vi "Copy .LLB to NI VeriStand dir.vi"(5 "Files Generated by Build":path[](array[path]), 6 "Top Level/Always Included VIs":path[](array[path]), 7 "Destination Path":path, 8 "error in (no error)":errorcluster, 9 "Target Name":string, 10 "Build Specification Name":string, 11 "Project Path":path) -> (0 "error out":errorcluster)   [LabVIEW 2015]
doc: "This VI is called after each run of a build specification. The VI will copy the generated LLB (Engine or System Explorer) into the VeriStand Custom Device folder (...\\Documents\\National Instruments\\NI VeriStand 2013...)."
uses:
  <vilib>/Utility/sysdir.llb/System Directory Type.ctl
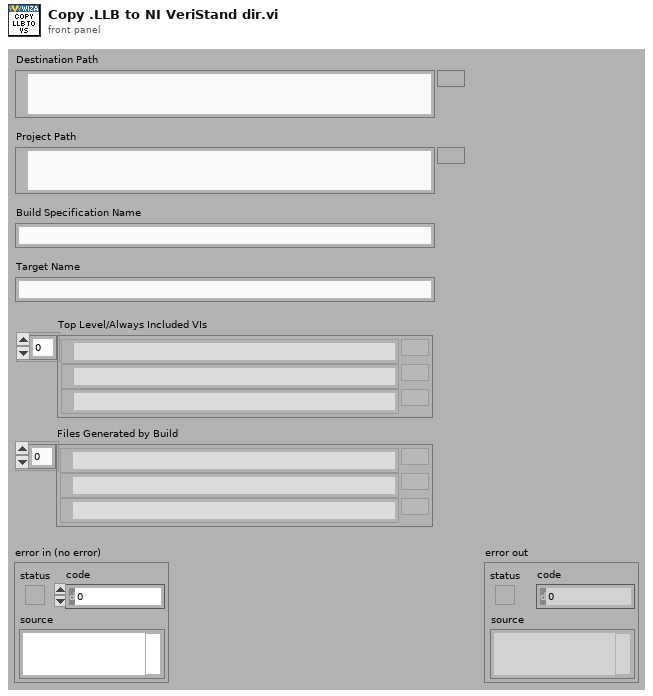
[diagram p1: front panel]
types:
  T1 = typedef "System Directory Type.ctl" = i32
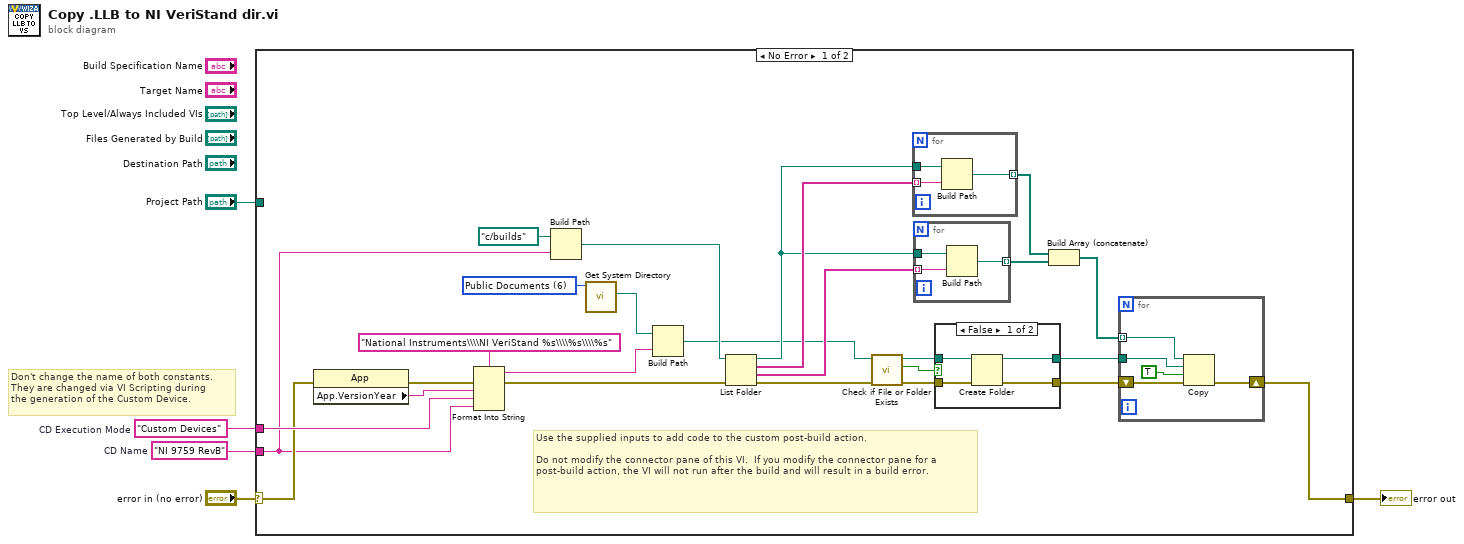
[diagram p0: block diagram]
diagram:
  w2 = "NI 9759 RevB"  # CD Name
  w3 = "Custom Devices"  # CD Execution Mode
  # "Don't change the name of both constants.\nThey are changed via VI Scripting during\nthe generation of the Custom Device."
  n1 = case shown="No Error" "error in (no error)" {
    selector: "error in (no error)" -> [w11 w49]
    tunnel: [w14 w49] -> w1
    tunnel: "Project Path" -> [_ _]
    tunnel: w3 -> [w12 _]
    tunnel: w2 -> [w9 _]
    frame No Error {
      w18 = T1 6 items=["User Home"=0, "User Desktop"=1, "User Documents"=2, "User Application Data"=3, "User Preferences"=4, "User Temporary"=5, "Public Documents"=6, "Public Application Data"=7, "Public Preferences"=8, "Public Cache"=13, "System Core Libraries"=9, "System Installed Libraries"=10, "Application Files"=11, "Boot Volume Root"=12] ("system directory type")
      # "Use the supplied inputs to add code to the custom post-build action.\n\nDo not modify the connector pane of this VI.  If you modify the connector pane for a post-build action, the VI will not run after the build and will result in a build error."
      n2 = property class="App"(error in=w11) -> (error out=w17:errorcluster, "App.VersionYear"=w16:string)  [unwired: 1 in, 1 out]
      n3 = Format Into String(format string="National Instruments\\\\NI VeriStand %s\\\\%s\\\\%s" ("name or relative path"), error in=w17, w16, w12, w9) -> (resulting string=w20:string, error out=w10:errorcluster)  [unwired: 1 in]
      n4 = Build Path(base path=path "c:/builds" ("name or relative path"), name or relative path=w9) -> (appended path=w22:path)
      n5 = call <vilib>:"Get System Directory.vi"("system directory type"=w18) -> ("system directory"=w19:path)  [unwired: 10 in]
      n6 = Build Path(base path=w19, name or relative path=w20) -> (appended path=w13:path)
      n7 = List Folder(path=w22, error in=w10) -> (path out=w24:path, filenames=w31:string[], folder names=w25:string[], error out=w21:errorcluster)  [unwired: 2 in]
      n8 = call <vilib>:"Check if File or Folder Exists.vi"("error in (no error)"=w21, "path"=w13) -> ("error out"=w26:errorcluster, "file or folder exists?"=w28:bool, "dup path"=w27:path)  [unwired: 7 in]
      n9 = for {
        tunnel: w31 -> [w47] mode=indexing
        tunnel: w24 -> [w48]
        tunnel: [w46] -> w30 mode=indexing
        n10 = Build Path(base path=w48, name or relative path=w47) -> (appended path=w46:path)
      }
      n11 = for {
        tunnel: w25 -> [w44] mode=indexing
        tunnel: w24 -> [w45]
        tunnel: [w43] -> w23 mode=indexing
        n12 = Build Path(base path=w45, name or relative path=w44) -> (appended path=w43:path)
      }
      n13 = case shown="False" w28 {
        tunnel: w27 -> [w35 w37]
        tunnel: w26 -> [w34 w36]
        tunnel: [w33 w37] -> w8
        tunnel: [w32 w36] -> w7
        frame False {
          n14 = Create Folder(path (use dialog)=w35, error in=w34) -> (created path=w33:path, error out=w32:errorcluster)  [unwired: 1 in, 1 out]
        }
        frame True {
        }
      }
      n15 = Build Array (concatenate)(w30, w23) -> (w29:path[])
      n16 = for {
        tunnel: w29 -> [w39] mode=indexing
        shift-right: [w40] -> w14
        shift-left: w7 -> [w41]
        tunnel: w8 -> [w38]
        n17 = Copy(8:w41, 9:TRUE ("overwrite (F)"), 10:w38, 11:w39) -> (0:w40:errorcluster)  [unwired: 1 in, 2 out]
      }
    }
    frame Error {
    }
  }
  "error out" <- w1
